vi "DATOS_EXCEL.vi"(7 "timestamp":dbl, 8 "Max RMS Ruedas":dbl[][](array[numeric]), 9 "Array TAGs 2":string[](array[string]), 10 "p_sp 2":dbl, 11 "p_tp 2":dbl) -> (0 "error out":errorcluster)   [LabVIEW 2015]
uses:
  <vilib>/Utility/file.llb/Write Delimited Spreadsheet (string).vi
panel:
  out "Array 2":string[][](array[string])
  out "Array":string[][](array[string])
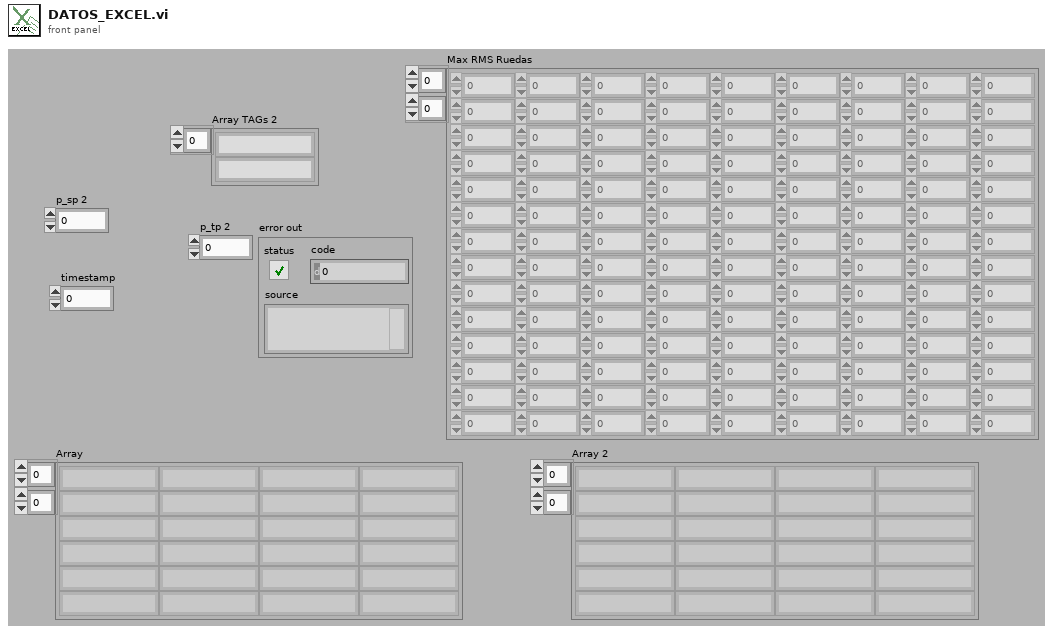
[diagram p1: front panel]
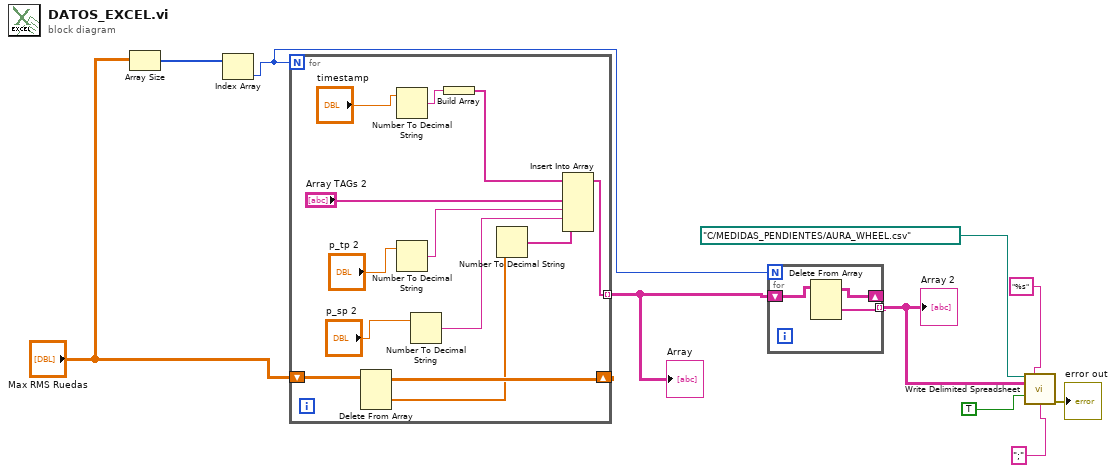
[diagram p0: block diagram]
diagram:
  n1 = Array Size(array="Max RMS Ruedas") -> (size(s)=w3:i32[])
  n2 = Index Array(array=w3) -> (element=w2:i32)  [unwired: 1 in]
  n3 = for {
    N: w2 -> [_]
    shift-right: [w23] -> _
    shift-left: "Max RMS Ruedas" -> [w16]
    tunnel: [w11] -> w5 mode=indexing
    n4 = Delete From Array(array=w16) -> (deleted portion=w15:dbl[], array with subset deleted=w23:dbl[][])  [unwired: 3 in]
    n5 = Number To Decimal String(number="timestamp") -> (decimal integer string=w13:string)  [unwired: 1 in]
    n6 = Number To Decimal String(number="p_tp 2") -> (decimal integer string=w20:string)  [unwired: 1 in]
    n7 = Number To Decimal String(number="p_sp 2") -> (decimal integer string=w21:string)  [unwired: 1 in]
    n8 = Build Array(w13) -> (w12:string[])
    n9 = Number To Decimal String(number=w15) -> (decimal integer string=w22:string[])  [unwired: 1 in]
    n10 = Insert Into Array(array=w12, new element #1="Array TAGs 2", new element #2=w20, new element #3=w21, new element #4=w22) -> (w11:string[])  [unwired: 1 in]
  }
  "Array" <- w5
  n11 = for {
    N: w2 -> [_]
    shift-right: [w25] -> _
    shift-left: w5 -> [w26]
    tunnel: [w24] -> w4 mode=indexing
    n12 = Delete From Array(array=w26) -> (deleted portion=w24:string[], array with subset deleted=w25:string[][])  [unwired: 3 in]
  }
  "Array 2" <- w4
  n13 = call-poly <vilib>:"Write Delimited Spreadsheet.vi"("file path (dialog if empty)"=path "C:/MEDIDAS_PENDIENTES/AURA_WHEEL.csv", "format (%s)"="%s" ("format (%.3f)"), "2D data"=w4, "append to file? (F)"=TRUE ("append to file? (new file:F)"), "delimiter (\\t)"=";" ("delimiter (\\t)")) -> ("error out"=→"error out":errorcluster)  [unwired: 9 in, 1 out]
